vi "ACT_Loop.vi"() -> ()   [LabVIEW 2020, in "Tube Wheel_ACT.lvlib"]
uses:
  Tube Wheel_ACT.lvlib
  Cluster_CMD_ACT_Data.ctl
  Type Defs/ENUM_TubeWheel_Mode.ctl
  Type Defs/ENUM_Tube Wheel CMD Positions.ctl
  Type Defs/Cluster_Tube Wheel Positions.ctl
  Shared Code/TypeDefs/ENUM_Tube Wheel Positions.ctl
  Shared Code/TypeDefs/Cluster_PID Gains.ctl
  ENUM_ACT_State.ctl
  <vilib>/Rock Robotics/WPI/MotorControl/WPI_MotorControlDeviceRef.ctl
  <vilib>/Rock Robotics/WPI/MotorControl/WPI_MotorControlType.ctl
  <vilib>/Rock Robotics/SystemInterfaces/DIO/FPGA_DIOPWMChannel.ctl
  <vilib>/Rock Robotics/WPI/PWM/WPI_PWMDeadband.ctl
  <vilib>/Rock Robotics/SystemInterfaces/DIO/FPGA_DIOChannel.ctl
  Support VIs/Absolute Encoder/Cluster_Absolute Encoder Ref.ctl
  <vilib>/Rock Robotics/SystemInterfaces/DutyCycle/FPGA_DutyCycleDevRef.ctl
  <vilib>/Rock Robotics/SystemInterfaces/DutyCycle/FPGA_DutyCycleIndex.ctl
  <vilib>/Rock Robotics/WPI/Counter/WPI_CounterDevRef.ctl
  <vilib>/Rock Robotics/SystemInterfaces/Counter/FPGA_CounterCtrSystemIndex.ctl
  ENUM_ACT_Action.ctl
  Shared Code/TypeDefs/Cluster_High-Low.ctl
  c4c8c652-40d9-430f-9271-bf9f3a6ec4c9.vi
  ba1a27d8-7cfb-4bdd-8bd7-cd7ea4f4c7ec.vi
  195b1e84-ccd7-4ca0-9bd4-16477e8a770f.vi
  82f0efda-27c2-462c-9bd9-b1e49375ea7b.vi
  f27dd756-8008-48f9-894a-7d8dfba90c72.vi
  63a73014-4d80-4d9e-ab4e-dbaa010192ad.vi
  <vilib>/Rock Robotics/WPI/MotorControl/WPI_MotorControlOpen VictorSP.vi
  RoboRIO Utilities/Global_STOP.vi
  Global_CMD_ACT_Data In.vi
  Feeder/Global_ACT_Data Out.vi
  Global_ACT_Data Out.vi
  <vilib>/Comparison/Equal/Equal Functor/Equal Functor.lvclass
  Feeder/Feeder_ACT.lvlib
panel:
  out "Wheel Count":i32
  in  "IZone":i32=70
  out "Time Mulitplyer Out":dbl
  out "PID Enabled Out":bool
  in  "PID Gains":T1={"P"=0.0015, "I"=0.0002, "D"=0.0, "F"=0.0} {"F" format="%#.8f"; "D" format="%#.8f"; "I" format="%#.8f"; "P" format="%#.8f"}
  out "Pusher Back":bool
  out "Output":dbl
  out "ERROR":i32
  in  "Min Output":dbl=0.08
  in  "Allowable Error":i32=2
  in  "Max Output":dbl=0.25
  out "@ target":bool
  out "Current Position":T2
  in  "Position Array":T3[](array[typedef])=[{"Positions"=enum."Tube Black B", "Count"=45}, {"Positions"=enum."Tube Red A", "Count"=214}, {"Positions"=enum."Tube Black F", "Count"=384}, {"Positions"=enum."Tube Red E", "Count"=555}, {"Positions"=enum."Tube Black D", "Count"=727}, {"Positions"=enum."Tube Red C", "Count"=894}]
  out "Input DBL Data":T4 {"Motor speed (0-1)" format="%.3g"}
  out "Wheel Position":i32
  out "Cycle Time (S)":dbl format="%.3g"
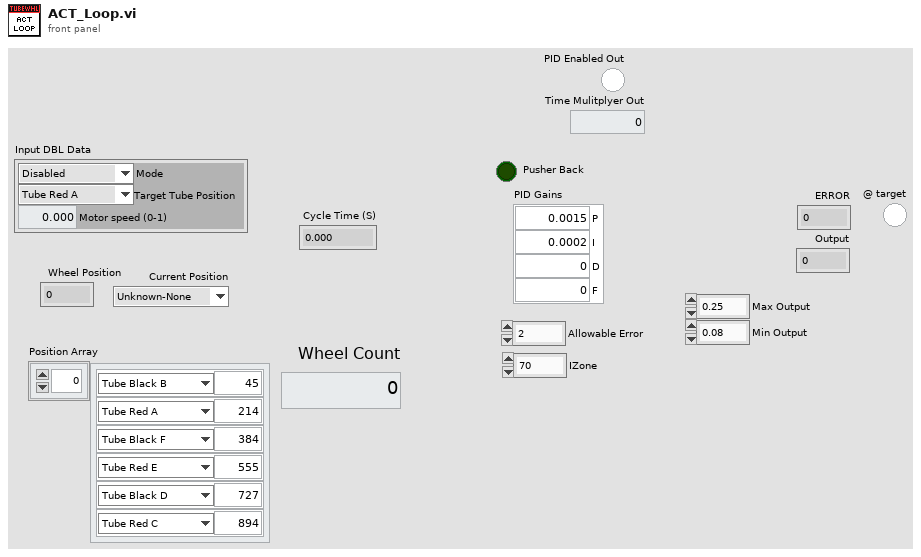
[diagram p1: front panel]
types:
  T1 = typedef "Cluster_PID Gains.ctl" = cluster{"P":dbl, "I":dbl, "D":dbl, "F":dbl}
  T2 = typedef "ENUM_Tube Wheel Positions.ctl" = enum16{"Unknown-None", "Tube Red A", "Tube Black B", "Tube Red C", "Tube Black D", "Tube Red E", "Tube Black F", "Load A-B", "Load B-C", "Load C-D", "Load D-E", "Load E-F", "Load F-A"}
  T3 = typedef "Cluster_Tube Wheel Positions.ctl" = cluster{"Positions":T2, "Count":i32}
  T4 = typedef "Tube Wheel_ACT.lvlib/Cluster_CMD_ACT_Data.ctl" = cluster{"Mode":T5, "Target Tube Position":T6, "Motor speed (0-1)":dbl}
  T5 = typedef "ENUM_TubeWheel_Mode.ctl" = enum16{"Disabled", "Manual Motor", "Select Positon"}
  T6 = typedef "ENUM_Tube Wheel CMD Positions.ctl" = enum16{"Tube Red A", "Tube Black B", "Tube Red C", "Tube Black D", "Tube Red E", "Tube Black F"}
  T7 = typedef "FPGA_DIOChannel.ctl" = enum8{"DIO 0", "DIO 1", "DIO 2", "DIO 3", "DIO 4", "DIO 5", "DIO 6", "DIO 7", "DIO 8", "DIO 9", "DIO MXP 0", "DIO MXP 1", "DIO MXP 2", "DIO MXP 3", "DIO MXP 4", "DIO MXP 5", "DIO MXP 6", "DIO MXP 7", "DIO MXP 8", "DIO MXP 9", "DIO MXP 10", "DIO MXP 11", "DIO MXP 12", "DIO MXP 13", "DIO MXP 14", "DIO MXP 15", "SPI Port CS1", "SPI Port CS2", "SPI Port CS3", "SPI Port MISO", "SPI Port MOSI", "Invalid"}
  T8 = typedef "Cluster_Absolute Encoder Ref.ctl" = cluster{"DutyCycleDevRef":T9, "CounterDevRef":T11}
  T9 = typedef "FPGA_DutyCycleDevRef.ctl" = cluster{"DevStatus":errorcluster, "DutyCycleIndex":T10}
  T10 = typedef "FPGA_DutyCycleIndex.ctl" = enum8{"DutyCycle 0", "DutyCycle 1", "DutyCycle 2", "DutyCycle 3", "DutyCycle 4", "DutyCycle 5", "DutyCycle 6", "DutyCycle 7", "Invalid"}
  T11 = typedef "WPI_CounterDevRef.ctl" = cluster{"DevStatus":errorcluster, "CntIndex":T12}
  T12 = typedef "FPGA_CounterCtrSystemIndex.ctl" = enum8{"Ctr 0", "Ctr 1", "Ctr 2", "Ctr 3", "Ctr 4", "Ctr 5", "Ctr 6", "Ctr 7", "Invalid"}
  T13 = typedef "FPGA_DIOPWMChannel.ctl" = enum8{"PWM 0", "PWM 1", "PWM 2", "PWM 3", "PWM 4", "PWM 5", "PWM 6", "PWM 7", "PWM 8", "PWM 9", "PWM MXP 0", "PWM MXP 1", "PWM MXP 2", "PWM MXP 3", "PWM MXP 4", "PWM MXP 5", "PWM MXP 6", "PWM MXP 7", "PWM MXP 8", "PWM MXP 9", "Invalid"}
  T14 = typedef "WPI_MotorControlDeviceRef.ctl" = cluster{"DeviceStatus":errorcluster, "Type":T15, "PWM":cluster{"PWM Channel":T13, "DeadBand":T16}, "CAN":cluster{"Device Number":u8, "SetOutput VI Ref":variant, "GetOutput VI Ref":variant, "Enable VI Ref":variant, "Disable VI Ref":variant, "Data":variant}, "Invert":bool, "DIO PWM":cluster{"PWM \"Enable\" Channel":T13, "DIOChannel":T7, "PWM Rate":dbl}}
  T15 = typedef "WPI_MotorControlType.ctl" = enum16{"PWM", "CAN", "DIO PWM"}
  T16 = typedef "WPI_PWMDeadband.ctl" = cluster{"Name":string, "maxPositivePwm":i32, "minPositivePwm":i32, "centerPwm":i32, "maxNegativePwm":i32, "minNegativePwm":i32, "angularRange":u16}
  T17 = typedef "Tube Wheel_ACT.lvlib/ENUM_ACT_State.ctl" = enum16{"Startup", "Stopping", "Moving to Positon", "Moving Manually", "Shutdown"}
  T18 = typedef "Tube Wheel_ACT.lvlib/ENUM_ACT_Action.ctl" = enum16{"No Action", "Reset Time", "Reset All", "MoveToPosition", "Stop", "Set Motor Speed Manually"}
  T19 = cluster{"Wheel Motor Ref":T14, "Wheel Encoder Ref":T8, "State":T17, "Previous State":T17, "Current Time":timestamp, "Previous Time":timestamp, "Start Time":timestamp, "Target Time (ms)":u32, "Cycle Time(S)":dbl, "ACT Input":T4, "Wheel Count":i32, "Motor Value":dbl, "Tube Positions":T2[], "Tube Counts":i32[], "Target Count":i32, "Current Position":T2, "At Target":bool, "Count Error":i32, "PPR":i32, "Min output":dbl, "Allowable Error":i32, "Stable Time":dbl, "At Target Time":dbl, "Pusher Back":bool}
  T20 = typedef "Cluster_High-Low.ctl" = cluster{"High":dbl, "Low":dbl}
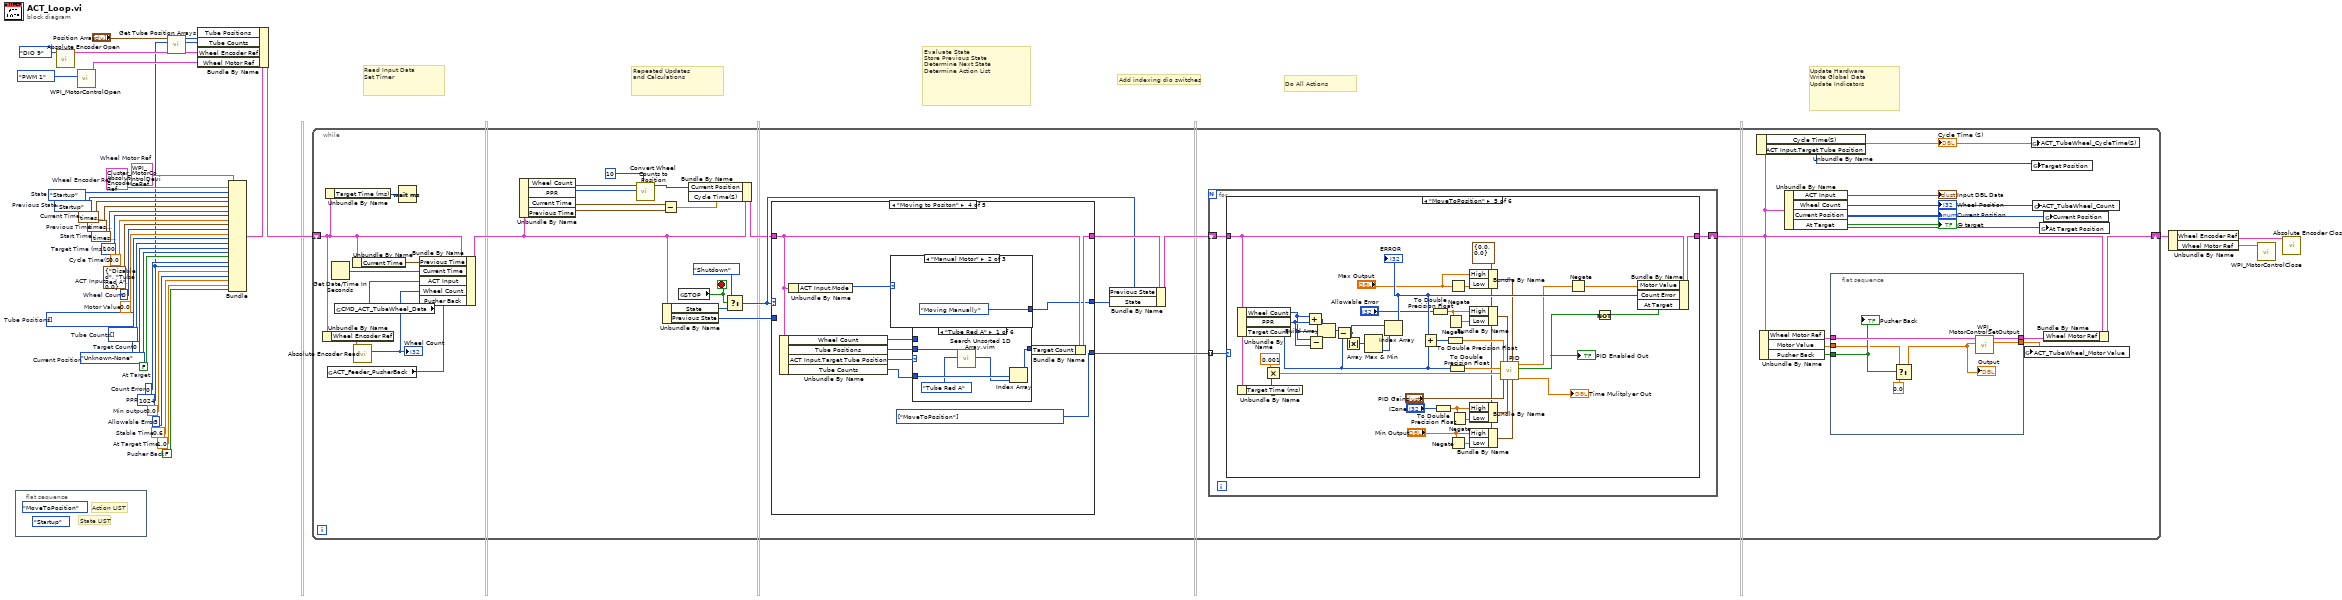
[diagram p0: block diagram]
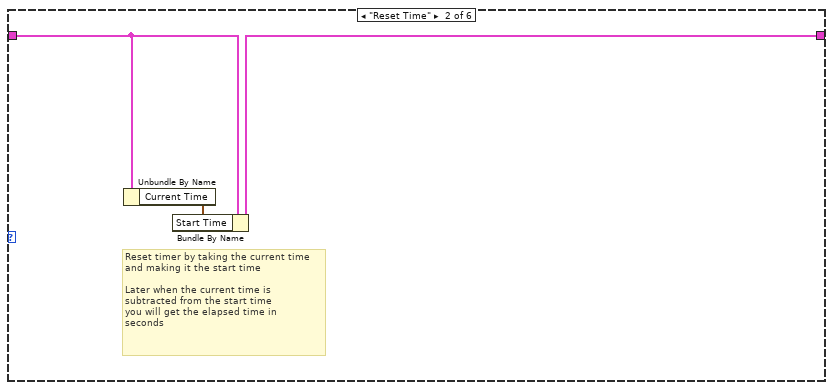
[diagram p3: hidden frame]
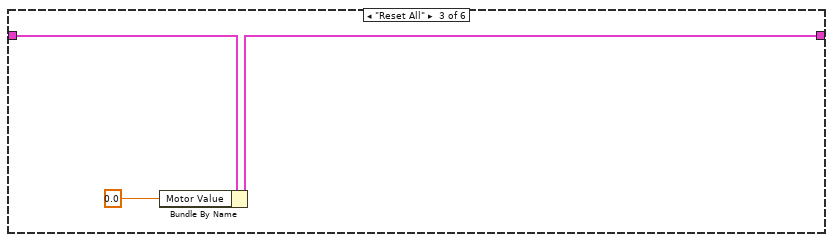
[diagram p4: hidden frame]
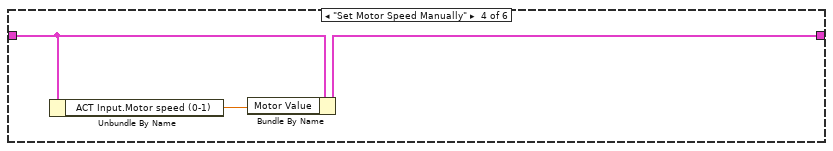
[diagram p5: hidden frame]
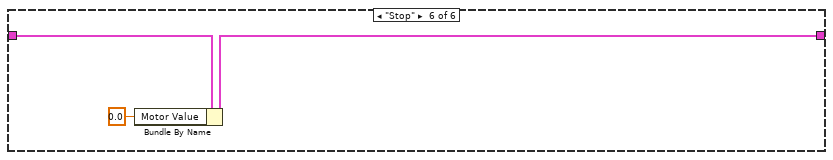
[diagram p6: hidden frame]
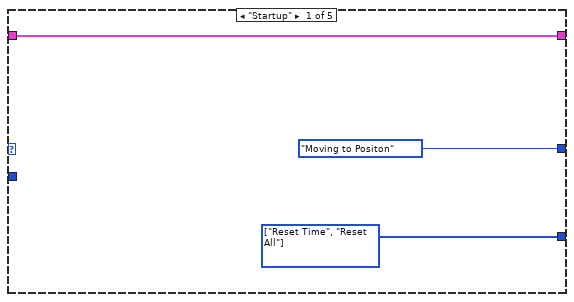
[diagram p7: hidden frame]
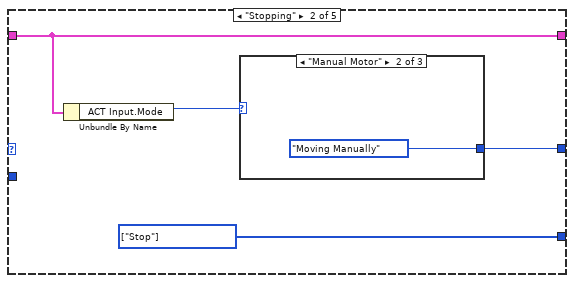
[diagram p8: hidden frame]
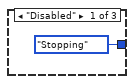
[diagram p9: hidden frame]
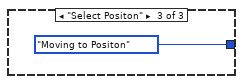
[diagram p10: hidden frame]
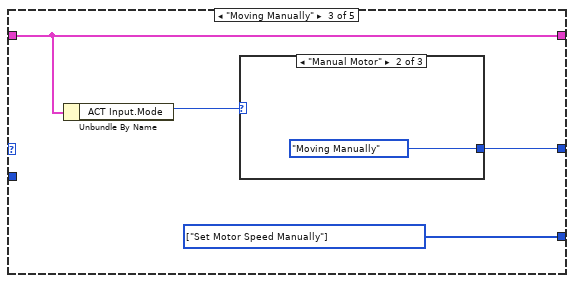
[diagram p11: hidden frame]
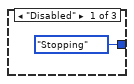
[diagram p12: hidden frame]
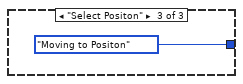
[diagram p13: hidden frame]
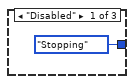
[diagram p14: hidden frame]
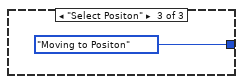
[diagram p15: hidden frame]
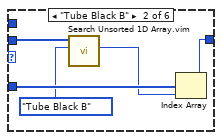
[diagram p16: hidden frame]
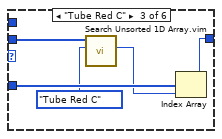
[diagram p17: hidden frame]
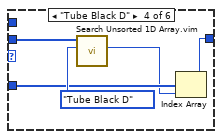
[diagram p18: hidden frame]
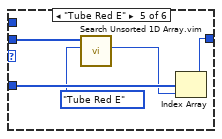
[diagram p19: hidden frame]
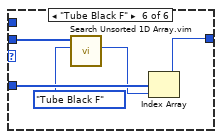
[diagram p20: hidden frame]
diagram:
  w1 = FALSE  # Pusher Back
  w2 = 1.0  # At Target Time
  w3 = 0.6  # Stable Time
  w5 = 0.0  # Min output
  w4 = 3  # Allowable Error
  w6 = 1024  # PPR
  w7 = 0  # Count Error
  w9 = FALSE  # At Target
  w10 = ENUM_Tube_Wheel_Positions."Unknown-None"  # Current Position
  w11 = 0  # Target Count
  w14 = i32[] []  # Tube Counts
  w15 = T2[] [] items=["Unknown-None", "Tube Red A", "Tube Black B", "Tube Red C", "Tube Black D", "Tube Red E", "Tube Black F", "Load A-B", "Load B-C", "Load C-D", "Load D-E", "Load E-F", "Load F-A"]  # Tube Positions
  w18 = T8 {"DutyCycleDevRef"={"DevStatus"={"status"=FALSE, "code"=0, "source"=""}, "DutyCycleIndex"=enum."DutyCycle 0"}, "CounterDevRef"={"DevStatus"={"status"=FALSE, "code"=0, "source"=""}, "CntIndex"=enum."Ctr 0"}}  # Wheel Encoder Ref
  w21 = 0.0  # Motor Value
  w24 = T14 {"DeviceStatus"={"status"=FALSE, "code"=0, "source"=""}, "Type"=enum."PWM", "PWM"={"PWM Channel"=enum."Invalid", "DeadBand"={"Name"="", "maxPositivePwm"=0, "minPositivePwm"=0, "centerPwm"=0, "maxNegativePwm"=0, "minNegativePwm"=0, "angularRange"=0}}, "CAN"={"Device Number"=0, "SetOutput VI Ref"=variant(refnum<vi> refnum), "GetOutput VI Ref"=variant(refnum<vi> refnum), "Enable VI Ref"=variant(refnum<vi> refnum), "Disable VI Ref"=variant(refnum<vi> refnum), "Data"=variant}, "Invert"=FALSE, "DIO PWM"={"PWM \"Enable\" Channel"=enum."Invalid", "DIOChannel"=enum."Invalid", "PWM Rate"=0.0}}  # Wheel Motor Ref
  w28 = 0.0  # Cycle Time(S)
  w29 = ENUM_ACT_State."Startup"  # Previous State
  w30 = timestamp(0 s since 1904-01-01)  # Previous Time
  w31 = u32 100  # Target Time (ms)
  w32 = 0  # Wheel Count
  w33 = T4 {"Mode"=enum."Disabled", "Target Tube Position"=enum."Tube Red A", "Motor speed (0-1)"=0.0}  # ACT Input
  w34 = timestamp(0 s since 1904-01-01)  # Start Time
  w35 = timestamp(0 s since 1904-01-01)  # Current Time
  w36 = ENUM_ACT_State."Startup"  # State
  # "Add indexing dio switches"
  # "Repeated Updates\nand Calculations"
  # "Read Input Data\nSet Timer"
  # "Evaluate State\nStore Previous State\nDetermine Next State\nDetermine Action List"
  # "Do All Actions"
  # "Update Hardware\nWrite Global Data\nUpdate Indicators"
  n1 = flat-sequence {
    frame #0 {
      (unwired) ENUM_ACT_State."Startup" ("State")
      (unwired) ENUM_ACT_Action."MoveToPosition" ("Action")
      # "State LIST"
      # "Action LIST"
    }
  }
  n2 = call "Absolute Encoder Open.vi"("Channel"=FPGA_DIOChannel."DIO 9") -> ("Cluster"=w17:T8)  [unwired: 9 in, 1 out]
  n3 = call-poly <vilib>:"WPI_MotorControlOpen.vi"("PWM Channel"=FPGA_DIOPWMChannel."PWM 1") -> ("MotorControlDeviceRef"=w23:T14)  [unwired: 9 in, 1 out]
  n4 = call "Get Tube Position Arrays.vi"("PPR"=w6, "Position Array"="Position Array") -> ("Counts"=w12:i32[], "Positons"=w13:T2[])  [unwired: 8 in]
  n5 = Bundle("Wheel Motor Ref"=w24, "Wheel Encoder Ref"=w18, "State"=w36, "Previous State"=w29, "Current Time"=w35, "Previous Time"=w30, "Start Time"=w34, "Target Time (ms)"=w31, "Cycle Time(S)"=w28, "ACT Input"=w33, "Wheel Count"=w32, "Motor Value"=w21, "Tube Positions"=w15, "Tube Counts"=w14, "Target Count"=w11, "Current Position"=w10, "At Target"=w9, "Count Error"=w7, "PPR"=w6, "Min output"=w5, "Allowable Error"=w4, "Stable Time"=w3, "At Target Time"=w2, "Pusher Back"=w1) -> (w26:T19)  [unwired: 1 in]
  n6 = Bundle By Name(cluster=w26, "Tube Positions"=w13, "Tube Counts"=w12, "Wheel Encoder Ref"=w17, "Wheel Motor Ref"=w23) -> (w25:T19)
  n7 = while {
    shift-right: [w54] -> w27
    shift-left: w25 -> [w50]
    stop <- w72 stop-if-true
    n8 = Unbundle By Name(w50) -> ("Wheel Encoder Ref"=w49:T8)
    n9 = Unbundle By Name(w50) -> ("Target Time (ms)"=w69:u32)
    n10 = global read "Global_ACT_Data Out.vi" "ACT_Feeder_PusherBack"() -> (w38:bool)
    n11 = Get Date/Time In Seconds() -> (seconds since 1Jan1904=w75:timestamp)
    n12 = global read "Global_CMD_ACT_Data In.vi" "CMD_ACT_TubeWheel_Data"() -> (w58:T4)
    n13 = Unbundle By Name(w50) -> ("Current Time"=w68:timestamp)
    n14 = call "Absolute Encoder Read.vi"("Cluster"=w49) -> ("Single Encoder Counts Out"=w39:i32)  [unwired: 4 in, 6 out]
    "Wheel Count" <- w39
    n15 = Wait (ms)(milliseconds to wait=w69) -> ()  [unwired: 1 out]
    n16 = Bundle By Name(cluster=w50, "Previous Time"=w68, "Current Time"=w75, "ACT Input"=w58, "Wheel Count"=w39, "Pusher Back"=w38) -> (w63:T19)
    n17 = Unbundle By Name(w63) -> ("Wheel Count"=w43:i32, "PPR"=w41:i32, "Current Time"=w64:timestamp, "Previous Time"=w65:timestamp)
    n18 = call "Convert Wheel Counts to Position.vi"("Count Tollerance"=10, "PPR"=w41, "Wheel Count"=w43) -> ("Current Positions Out"=w44:T2)  [unwired: 8 in]
    n19 = Subtract(x=w64, y=w65) -> (x-y=w61:dbl)
    n20 = Unbundle By Name(w63) -> ("State"=w70:T17, "Previous State"=w67:T17)
    n21 = global read "Global_STOP.vi" "STOP"() -> (w72:bool)
    n22 = Bundle By Name(cluster=w63, "Current Position"=w44, "Cycle Time(S)"=w61) -> (w62:T19)
    n23 = Select(t=ENUM_ACT_State."Shutdown" ("State"), s=w72, f=w70) -> (s? t:f=w66:T17)
    n24 = case shown="\"Moving to Positon\"" w66 {
      tunnel: w62 -> [w140 w142 w149 w157 w200]
      tunnel: [w140 w142 w149 w161 w200] -> w73
      tunnel: [w139 w141 w148 w159 w199] -> w60
      tunnel: w67 -> [_ _ _ _ _]
      tunnel: [ENUM_ACT_State."Moving to Positon" ("State") w143 w150 w155 ENUM_ACT_State."Shutdown" ("State")] -> w40
      frame "Startup" {
        w139 = T18[] [enum."Reset Time", enum."Reset All"] items=["No Action", "Reset Time", "Reset All", "MoveToPosition", "Stop", "Set Motor Speed Manually"] ("Actions")
      }
      frame "Stopping" {
        w141 = T18[] [enum."Stop"] items=["No Action", "Reset Time", "Reset All", "MoveToPosition", "Stop", "Set Motor Speed Manually"] ("Actions")
        n25 = Unbundle By Name(w142) -> ("ACT Input.Mode"=w144:T5)
        n26 = case shown="\"Manual Motor\"" w144 {
          tunnel: [ENUM_ACT_State."Stopping" ("State") ENUM_ACT_State."Moving Manually" ("State") ENUM_ACT_State."Moving to Positon" ("State")] -> w143
          frame "Disabled" {
          }
          frame "Manual Motor" {
          }
          frame "Select Positon" {
          }
        }
      }
      frame "Moving Manually" {
        w148 = T18[] [enum."Set Motor Speed Manually"] items=["No Action", "Reset Time", "Reset All", "MoveToPosition", "Stop", "Set Motor Speed Manually"] ("Actions")
        n27 = Unbundle By Name(w149) -> ("ACT Input.Mode"=w151:T5)
        n28 = case shown="\"Manual Motor\"" w151 {
          tunnel: [ENUM_ACT_State."Stopping" ("State") ENUM_ACT_State."Moving Manually" ("State") ENUM_ACT_State."Moving to Positon" ("State")] -> w150
          frame "Disabled" {
          }
          frame "Manual Motor" {
          }
          frame "Select Positon" {
          }
        }
      }
      frame "Moving to Positon" {
        w159 = T18[] [enum."MoveToPosition"] items=["No Action", "Reset Time", "Reset All", "MoveToPosition", "Stop", "Set Motor Speed Manually"] ("Actions")
        n29 = Unbundle By Name(w157) -> ("Wheel Count"=w158:i32, "Tube Positions"=w164:T2[], "ACT Input.Target Tube Position"=w163:T6, "Tube Counts"=w162:i32[])
        n30 = Unbundle By Name(w157) -> ("ACT Input.Mode"=w156:T5)
        n31 = case shown="\"Manual Motor\"" w156 {
          tunnel: [ENUM_ACT_State."Stopping" ("State") ENUM_ACT_State."Moving Manually" ("State") ENUM_ACT_State."Moving to Positon" ("State")] -> w155
          frame "Disabled" {
          }
          frame "Manual Motor" {
          }
          frame "Select Positon" {
          }
        }
        n32 = case shown="\"Tube Red A\"" w163 {
          tunnel: w164 -> [w170 w175 w180 w186 w190 w195]
          tunnel: w162 -> [w172 w177 w182 w184 w192 w197]
          tunnel: [w171 w176 w181 w187 w191 w196] -> w160
          tunnel: w158 -> [_ _ _ _ _ _]
          frame "Tube Red A" {
            n33 = call "Search Unsorted 1D Array.vim"("element"=ENUM_Tube_Wheel_Positions."Tube Red A" ("Tube Wheel Positions"), "unsorted 1D array"=w170) -> ("index of element"=w168:i32)  [unwired: 9 in]
            n34 = Index Array(array=w172, index=w168) -> (element=w171:i32)
          }
          frame "Tube Black B" {
            n35 = call "Search Unsorted 1D Array.vim"("element"=ENUM_Tube_Wheel_Positions."Tube Black B" ("Tube Wheel Positions"), "unsorted 1D array"=w175) -> ("index of element"=w173:i32)  [unwired: 9 in]
            n36 = Index Array(array=w177, index=w173) -> (element=w176:i32)
          }
          frame "Tube Red C" {
            n37 = call "Search Unsorted 1D Array.vim"("element"=ENUM_Tube_Wheel_Positions."Tube Red C" ("Tube Wheel Positions"), "unsorted 1D array"=w180) -> ("index of element"=w178:i32)  [unwired: 9 in]
            n38 = Index Array(array=w182, index=w178) -> (element=w181:i32)
          }
          frame "Tube Black D" {
            n39 = call "Search Unsorted 1D Array.vim"("element"=ENUM_Tube_Wheel_Positions."Tube Black D" ("Tube Wheel Positions"), "unsorted 1D array"=w186) -> ("index of element"=w183:i32)  [unwired: 9 in]
            n40 = Index Array(array=w184, index=w183) -> (element=w187:i32)
          }
          frame "Tube Red E" {
            n41 = call "Search Unsorted 1D Array.vim"("element"=ENUM_Tube_Wheel_Positions."Tube Red E" ("Tube Wheel Positions"), "unsorted 1D array"=w190) -> ("index of element"=w188:i32)  [unwired: 9 in]
            n42 = Index Array(array=w192, index=w188) -> (element=w191:i32)
          }
          frame "Tube Black F" {
            n43 = call "Search Unsorted 1D Array.vim"("element"=ENUM_Tube_Wheel_Positions."Tube Black F" ("Tube Wheel Positions"), "unsorted 1D array"=w195) -> ("index of element"=w193:i32)  [unwired: 9 in]
            n44 = Index Array(array=w197, index=w193) -> (element=w196:i32)
          }
        }
        n45 = Bundle By Name(cluster=w157, "Target Count"=w160) -> (w161:T19)
      }
      frame "Shutdown" {
        w199 = T18[] [enum."Reset All"] items=["No Action", "Reset Time", "Reset All", "MoveToPosition", "Stop", "Set Motor Speed Manually"] ("Actions")
      }
    }
    n46 = Bundle By Name(cluster=w73, "Previous State"=w66, "State"=w40) -> (w74:T19)
    n47 = for {
      tunnel: w60 -> [w85] mode=indexing
      shift-right: [w84] -> w55
      shift-left: w74 -> [w83]
      n48 = case shown="\"MoveToPosition\"" w85 {
        tunnel: w83 -> [w86 w89 w92 w94 w125 w136]
        tunnel: [w86 w88 w91 w95 w134 w137] -> w84
        frame "No Action" {
        }
        frame "Reset Time" {
          # "Reset timer by taking the current time\nand making it the start time\n\nLater when the current time is \nsubtracted from the start time\nyou will get the elapsed time in \nseconds"
          n49 = Unbundle By Name(w89) -> ("Current Time"=w87:timestamp)
          n50 = Bundle By Name(cluster=w89, "Start Time"=w87) -> (w88:T19)
        }
        frame "Reset All" {
          n51 = Bundle By Name(cluster=w92, "Motor Value"=0.0 ("FG Write Value")) -> (w91:T19)
        }
        frame "Set Motor Speed Manually" {
          n52 = Unbundle By Name(w94) -> ("ACT Input.Motor speed (0-1)"=w93:dbl)
          n53 = Bundle By Name(cluster=w94, "Motor Value"=w93) -> (w95:T19)
        }
        frame "MoveToPosition" {
          w97 = T20 {"High"=0.0, "Low"=0.0} ("High Low")
          n54 = Unbundle By Name(w125) -> ("Wheel Count"=w132:i32, "PPR"=w133:i32, "Target Count"=w121:i32)
          n55 = Unbundle By Name(w125) -> ("Target Time (ms)"=w123:u32)
          n56 = Multiply(x=0.001 ("y"), y=w123) -> (x*y=w122:dbl)
          n57 = Add(x=w132, y=w133) -> (x+y=w131:i32)
          n58 = Subtract(x=w132, y=w133) -> (x-y=w130:i32)
          n59 = Build Array(w131, w132, w130) -> (w129:i32[])
          n60 = Subtract(x=w129, y=w121) -> (x-y=w126:i32[])
          n61 = Absolute Value(x=w126) -> (abs(x)=w128:i32[])
          n62 = Array Max & Min(array=w128) -> (min index (indices)=w127:i32)  [unwired: 3 out]
          n63 = Index Array(array=w126, index=w127) -> (element=w120:i32)
          "ERROR" <- w120
          n64 = Add(x=w120, y=w121) -> (x+y=w119:i32)
          n65 = To Double Precision Float(number="Allowable Error") -> (double precision float=w103:dbl)
          n66 = To Double Precision Float(number="IZone") -> (double precision float=w99:dbl)
          n67 = Negate(x=w103) -> (-x=w104:dbl)
          n68 = To Double Precision Float(number=w119) -> (double precision float=w114:dbl)
          n69 = To Double Precision Float(number=w121) -> (double precision float=w113:dbl)
          n70 = Negate(x="Max Output") -> (-x=w108:dbl)
          n71 = Negate(x="Min Output") -> (-x=w110:dbl)
          n72 = Negate(x=w99) -> (-x=w101:dbl)
          n73 = Bundle By Name(cluster=w97, "High"="Max Output", "Low"=w108) -> (w107:T20)
          n74 = Bundle By Name(cluster=w97, "High"=w103, "Low"=w104) -> (w106:T20)
          n75 = Bundle By Name(cluster=w97, "High"=w99, "Low"=w101) -> (w102:T20)
          n76 = Bundle By Name(cluster=w97, "High"="Min Output", "Low"=w110) -> (w112:T20)
          n77 = call "PID.vi"("Min Output"=w112, "Max Output"=w107, "Error I Zone"=w102, "Acceptable Error"=w106, "PID Gains"="PID Gains", "Target Cycle Time(S)"=w122, "Setpoint"=w113, "Process Variable"=w114) -> ("Time Mulitplyer Out"=→"Time Mulitplyer Out":dbl, "PID Enabled Out"=w117:bool, "Output Out"=w118:dbl)  [unwired: 1 out]
          "PID Enabled Out" <- w117
          n78 = Negate(x=w118) -> (-x=w98:dbl)
          n79 = Not(x=w117) -> (.not. x?=w116:bool)
          n80 = Bundle By Name(cluster=w125, "Motor Value"=w98, "Count Error"=w120, "At Target"=w116) -> (w134:T19)
        }
        frame "Stop" {
          n81 = Bundle By Name(cluster=w136, "Motor Value"=0.0) -> (w137:T19)
        }
      }
    }
    n82 = Unbundle By Name(w55) -> ("Cycle Time(S)"=w53:dbl, "ACT Input.Target Tube Position"=w47:T6)
    "Cycle Time (S)" <- w53
    n83 = Unbundle By Name(w55) -> ("Wheel Motor Ref"=w57:T14, "Motor Value"=w52:dbl, "Pusher Back"=w37:bool)
    n84 = Unbundle By Name(w55) -> ("ACT Input"=→"Input DBL Data":T4, "Wheel Count"=w48:i32, "Current Position"=w46:T2, "At Target"=w45:bool)
    "Wheel Position" <- w48
    "Current Position" <- w46
    "@ target" <- w45
    n85 = flat-sequence {
      tunnel: w57 -> [w81]
      tunnel: [w82] -> w56
      tunnel: w52 -> [w77]
      tunnel: [w80] -> w51
      tunnel: w37 -> [w79]
      frame #0 {
        n86 = Select(t=w77, s=w79, f=0.0) -> (s? t:f=w78:dbl)
        "Output" <- w78
        n87 = call <vilib>:"WPI_MotorControlSetOutput.vi"("Output"=w78, "MotorControlDevRef"=w81) -> ("Motor Output"=w80:dbl, "MotorControlDevRef"=w82:T14)  [unwired: 7 in, 1 out]
        "Pusher Back" <- w79
      }
    }
    n88 = global write "Global_ACT_Data Out.vi" "ACT_TubeWheel_Motor Value"(w51) -> ()
    n89 = global write "Global_ACT_Data Out.vi" "ACT_TubeWheel_CycleTime(S)"(w53) -> ()
    n90 = global write "Global_ACT_Data Out.vi" "Target Position"(w47) -> ()
    n91 = global write "Global_ACT_Data Out.vi" "ACT_TubeWheel_Count"(w48) -> ()
    n92 = global write "Global_ACT_Data Out.vi" "At Target Position"(w45) -> ()
    n93 = global write "Global_ACT_Data Out.vi" "Current Position"(w46) -> ()
    n94 = Bundle By Name(cluster=w55, "Wheel Motor Ref"=w56) -> (w54:T19)
  }
  n95 = Unbundle By Name(w27) -> ("Wheel Encoder Ref"=w20:T8, "Wheel Motor Ref"=w19:T14)
  n96 = call <vilib>:"WPI_MotorControlClose.vi"("MotorControlDevRef"=w19) -> ()  [unwired: 10 in, 1 out]
  n97 = call "Absolute Encoder Close.vi"("Cluster"=w20) -> ()  [unwired: 11 in]
